vi "RFC5322 DateString to Timestamp.vi"(11 "RFC5322 Date String":string) -> (1 "valid?":bool, 2 "UTC Time Offset":T1=enum."UTC-00:00", 3 "Timestamp":timestamp)   [LabVIEW 2018]
uses:
  <vilib>/LabVIEW Open Source Project/Epoch Date & Time/UTC Offsets -- enum.ctl
  <vilib>/LabVIEW Open Source Project/Epoch Date & Time/formatter.rfc5322/RFC5322 Months -- enum.ctl
  <vilib>/Utility/miscctls.llb/LVDateTimeRec.ctl
  <vilib>/regexp/Match Regular Expression.xnode
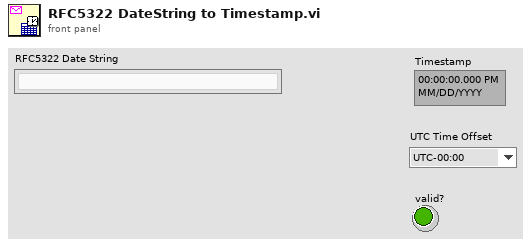
[diagram p1: front panel]
types:
  T1 = typedef "UTC Offsets -- enum.ctl" = enum16{"UTC-12:00", "UTC-11:00", "UTC-10:00", "UTC-09:30", "UTC-09:00", "UTC-08:00", "UTC-07:00", "UTC-06:00", "UTC-05:00", "UTC-04:00", "UTC-03:30", "UTC-03:00", "UTC-02:00", "UTC-01:00", "UTC-00:00", "UTC+00:00", "UTC+01:00", "UTC+02:00", "UTC+03:00", "UTC+03:30", "UTC+04:00", "UTC+04:30", "UTC+05:00", "UTC+05:30", "UTC+05:45", "UTC+06:00", "UTC+06:30", "UTC+07:00", "UTC+08:00", "UTC+08:45", "UTC+09:00", "UTC+09:30", "UTC+10:00", "UTC+10:30", "UTC+11:00", "UTC+12:00", "UTC+12:45", "UTC+13:00", "UTC+14:00"}
  T2 = typedef "RFC5322 Months -- enum.ctl" = enum16{"Jan", "Feb", "Mar", "Apr", "May", "Jun", "Jul", "Aug", "Sep", "Oct", "Nov", "Dec"}
  T3 = typedef "LVDateTimeRec.ctl" = cluster{"fractional second":dbl, "second":i32, "minute":i32, "hour":i32, "day of month":i32, "month":i32, "year":i32, "day of week":i32, "day of year":i32, "DST":i32}
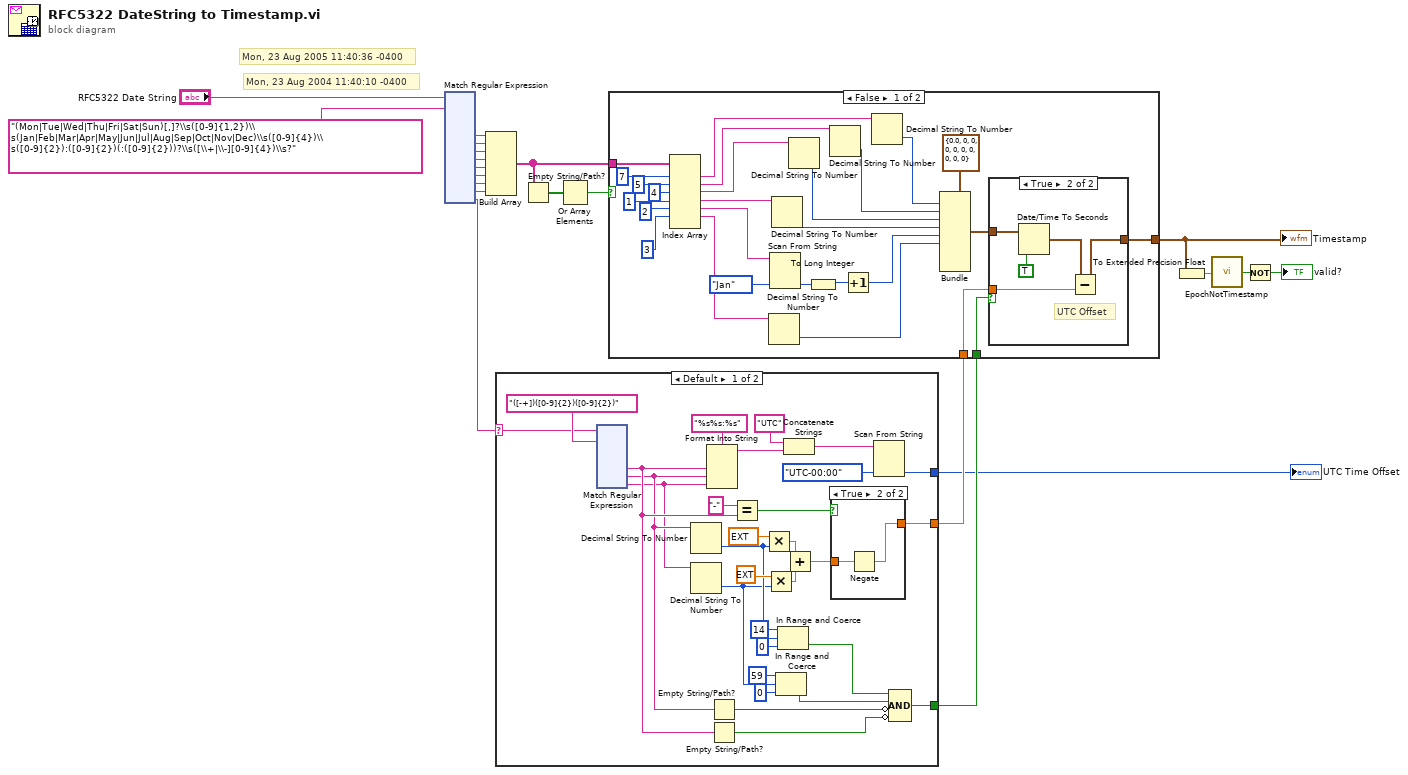
[diagram p0: block diagram]
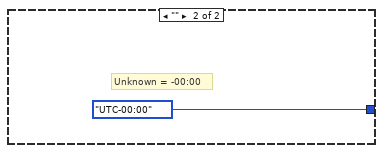
[diagram p3: hidden frame]
diagram:
  # "Mon, 23 Aug 2004 11:40:10 -0400"
  # "Mon, 23 Aug 2005 11:40:36 -0400"
  n1 = xnode "Match Regular Expression"("input string"="RFC5322 Date String", "regular expression"="(Mon|Tue|Wed|Thu|Fri|Sat|Sun)[,]?\\s([0-9]{1,2})\\s(Jan|Feb|Mar|Apr|May|Jun|Jul|Aug|Sep|Oct|Nov|Dec)\\s([0-9]{4})\\s([0-9]{2}):([0-9]{2})(:([0-9]{2}))?\\s([\\+|\\-][0-9]{4})\\s?") -> ("submatch 1"=w18:string, "submatch 2"=w17:string, "submatch 3"=w16:string, "submatch 4"=w15:string, "submatch 5"=w14:string, "submatch 6"=w13:string, "submatch 7"=w12:string, "submatch 8"=w11:string, "submatch 9"=w2:string)  [unwired: 4 in, 5 out]
  n2 = Build Array(w18, w17, w16, w15, w14, w13, w12, w11) -> (w1:string[])
  n3 = case shown="Default" w2 {
    selector: w2 -> [w27 _]
    tunnel: [w50 UTC_Offsets_--_enum."UTC-00:00" ("UTC Time Offset")] -> w4
    tunnel: [w40 _] -> w7
    tunnel: [w38 _] -> w6
    frame Default {
      n4 = xnode "Match Regular Expression"("input string"=w27, "regular expression"="([-+])([0-9]{2})([0-9]{2})") -> ("submatch 1"=w26:string, "submatch 2"=w25:string, "submatch 3"=w24:string)  [unwired: 4 in, 5 out]
      n5 = Decimal String To Number(string=w25) -> (number=w37:i32)  [unwired: 2 in, 1 out]
      n6 = Decimal String To Number(string=w24) -> (number=w31:i32)  [unwired: 2 in, 1 out]
      n7 = Format Into String(format string="%s%s:%s", w26, w25, w24) -> (resulting string=w22:string)  [unwired: 2 in, 1 out]
      n8 = Empty String/Path?(string/path=w25) -> (empty?=w39:bool)
      n9 = Empty String/Path?(string/path=w26) -> (empty?=w28:bool)
      n10 = Equal?(x="-" ("y"), y=w26) -> (x = y?=w41:bool)
      n11 = Multiply(x=ext 3600.0, y=w37) -> (x*y=w45:ext)
      n12 = Multiply(x=ext 60.0, y=w31) -> (x*y=w44:ext)
      n13 = In Range and Coerce(upper limit=59, x=w31, lower limit=0) -> (In Range?=w30:bool)  [unwired: 1 out]
      n14 = In Range and Coerce(upper limit=14, x=w37, lower limit=0) -> (In Range?=w34:bool)  [unwired: 1 out]
      n15 = Concatenate Strings("UTC" ("format string"), w22) -> (w49:string)
      n16 = Add(x=w45, y=w44) -> (x+y=w43:ext)
      n17 = case shown="True" w41 {
        tunnel: w43 -> [w170 w172]
        tunnel: [w170 w171] -> w40
        frame False {
        }
        frame True {
          n18 = Negate(x=w172) -> (-x=w171:ext)
        }
      }
      n19 = Scan From String(input string=w49, default 1=UTC_Offsets_--_enum."UTC-00:00" ("UTC Time Offset")) -> (output 1=w50:T1)  [unwired: 3 in, 3 out]
      n20 = Compound Arithmetic op=AND(w34, w30, invert w39, invert w28) -> (w38:bool)
    }
    frame "" {
      # "Unknown = -00:00"
    }
  }
  "UTC Time Offset" <- w4
  n21 = Empty String/Path?(string/path=w1) -> (empty?=w10:bool[])
  n22 = Or Array Elements(Boolean array=w10) -> (logical OR=w9:bool)
  n23 = case shown="False" w9 {
    tunnel: [w200 _] -> w3
    tunnel: w1 -> [w195 _]
    tunnel: w7 -> [w197 _]
    tunnel: w6 -> [w196 _]
    frame False {
      n24 = Index Array(array=w195, index #1=7 ("index"), index #2=5 ("index"), index #3=4 ("index"), index #4=1 ("index"), index #5=2 ("index"), index #6=3 ("index")) -> (element #1=w193:string, element #2=w189:string, element #3=w188:string, element #4=w185:string, element #5=w181:string, element #6=w175:string)  [unwired: 1 in, 1 out]
      n25 = Decimal String To Number(string=w175) -> (number=w174:i32)  [unwired: 2 in, 1 out]
      n26 = Scan From String(input string=w181, default 1=RFC5322_Months_--_enum."Jan") -> (output 1=w179:T2)  [unwired: 3 in, 3 out]
      n27 = Decimal String To Number(string=w185) -> (number=w183:i32)  [unwired: 2 in, 1 out]
      n28 = Decimal String To Number(string=w188) -> (number=w190:i32)  [unwired: 2 in, 1 out]
      n29 = To Long Integer(number=w179) -> (32bit integer=w178:i32)
      n30 = Decimal String To Number(string=w189) -> (number=w191:i32)  [unwired: 2 in, 1 out]
      n31 = Increment(x=w178) -> (x+1=w177:i32)
      n32 = Decimal String To Number(string=w193) -> (number=w192:i32)  [unwired: 2 in, 1 out]
      n33 = Bundle(cluster=T3 {"fractional second"=0.0, "second"=0, "minute"=0, "hour"=0, "day of month"=0, "month"=0, "year"=0, "day of week"=0, "day of year"=0, "DST"=0} ("date time rec"), "second"=w192, "minute"=w191, "hour"=w190, "day of month"=w183, "month"=w177, "year"=w174) -> (w198:T3)  [unwired: 4 in]
      n34 = case shown="True" w196 {
        tunnel: w198 -> [_ w204]
        tunnel: w197 -> [_ w203]
        tunnel: [_ w202] -> w200
        frame False {
        }
        frame True {
          # "UTC Offset"
          n35 = Date/Time To Seconds(1:TRUE ("is UTC (F)"), 2:w204) -> (0:w201:timestamp)
          n36 = Subtract(x=w201, y=w203) -> (x-y=w202:timestamp)
        }
      }
    }
    frame True {
    }
  }
  "Timestamp" <- w3
  n37 = To Extended Precision Float(1:w3) -> (0:w20:ext)
  n38 = call <vilib>:"EpochNotTimestamp.vi"("Epoch Time"=w20) -> ("Not a Timestamp?"=w21:bool)  [unwired: 8 in]
  n39 = Not(x=w21) -> (.not. x?=→"valid?":bool)
